vi "Calculate Feedforward.vi"() -> ()   [LabVIEW 2015]
uses:
  <vilib>/Rock Robotics/WPI/CAN/TalonSRX/WPI_CANTalonSRX_APIControlMode.ctl
  <vilib>/Rock Robotics/WPI/MotorControl/WPI_MotorControlOpenCANTalonSRX.vi
panel:
  in  "Counts per rev":i32
  in  "Device Number":i32
  in  "stop":bool
  in  "Start":bool
  in  "size of averaging array":i32
  in  "Deadzone":dbl format="%#_13g"
  out "Feedforward":dbl
  out "Applied Throttle":dbl
  out "Sensor Velocity":dbl
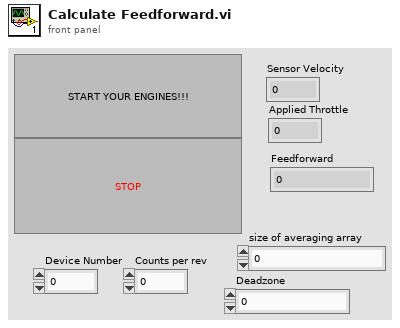
[diagram p1: front panel]
types:
  T1 = typedef "WPI_CANTalonSRX_APIControlMode.ctl" = enum8{"Percent VBus", "Speed", "Position", "Slave", "Unchanged / Invalid", "Voltage Compensation", "Current", "Motion Profile"}
  T2 = typedef "WPI_MotorControlDeviceRef.ctl" = cluster{"DeviceStatus":errorcluster, "Type":T3, "PWM":cluster{"PWM Channel":T4, "DeadBand":T5}, "CAN":cluster{"Device Number":u8, "Control Mode":T6, "Semaphore":T7, "Max Vout":dbl, "TalonSRX Control Mode":T1}, "Invert":bool}
  T3 = typedef "WPI_MotorControlType.ctl" = enum16{"PWM", "CAN", "CANTalonSRX"}
  T4 = typedef "FPGA_DIOPWMChannel.ctl" = enum8{"PWM 0", "PWM 1", "PWM 2", "PWM 3", "PWM 4", "PWM 5", "PWM 6", "PWM 7", "PWM 8", "PWM 9", "PWM MXP 0", "PWM MXP 1", "PWM MXP 2", "PWM MXP 3", "PWM MXP 4", "PWM MXP 5", "PWM MXP 6", "PWM MXP 7", "PWM MXP 8", "PWM MXP 9", "Invalid"}
  T5 = typedef "WPI_PWMDeadband.ctl" = cluster{"Name":string, "maxPositivePwm":i32, "minPositivePwm":i32, "centerPwm":i32, "maxNegativePwm":i32, "minNegativePwm":i32, "angularRange":u16}
  T6 = typedef "WPI_CANJaguar_ControlMode.ctl" = enum8{"Percent VBus", "Current", "Speed", "Position", "Voltage"}
  T7 = typedef "Semaphore RefNum" = refnum<k1>
  T8 = typedef "WPI_CANTalonSRX_GlobalStatus.ctl" = cluster{"Applied Throttle":dbl, "Module Enabled":bool, "CAN Error":errorcluster, "Closed Loop Error":dbl, "Forward Limit Switch Closed":bool, "Reverse Limit Switch Closed":bool, "Sensor Position":dbl, "Sensor Velocity":dbl, "Current":dbl, "Sticky Fault - Over Temp":bool, "Sticky Fault - Under Voltage":bool, "Sticky Fault - Forward Limit":bool, "Sticky Fault - Reverse Limit":bool, "Sticky Fault - Forward Soft Limit":bool, "Sticky Fault - Reverse Soft Limit":bool, "Brake is Enabled":bool, "Encoder Position":dbl, "Encoder Velocity":dbl, "Encoder Index Count":dbl, "Encoder A Pin State":bool, "Encoder B Pin State":bool, "Encoder Index Pin State":bool, "Analog In":dbl, "Analog In Velocity":dbl, "Temperature (C)":dbl, "Battery Voltage":dbl, "Control 5 Is Supported":bool, "Current Profile Slot Select":dbl, "Pos Div 8":bool, "Vel Div 4":bool, "Pulse Width Position":i32, "Pulse Width Velocity":i32, "Pulse Width Rise To Rise (us)":i32, "Pulse Width Rise To Fall (us)":i32, "Mot Prof Active Is Under Run":bool, "Mot Prof Active Has Under Run":bool, "Mot Prof Active Is Last":bool, "Mot Prof Active Velocity Only":bool, "Mot Prof Active Is Valid":bool, "Mot Prof Buffer Is Full":bool, "Mot Prof Active Profile Slot Select":i32, "Mot Prof NextID":i32, "Mot Prof Count":i32, "Mot Prof Active Velocity":dbl, "Mot Prof Active Position":dbl, "Mot Prof Output Enable":i32}
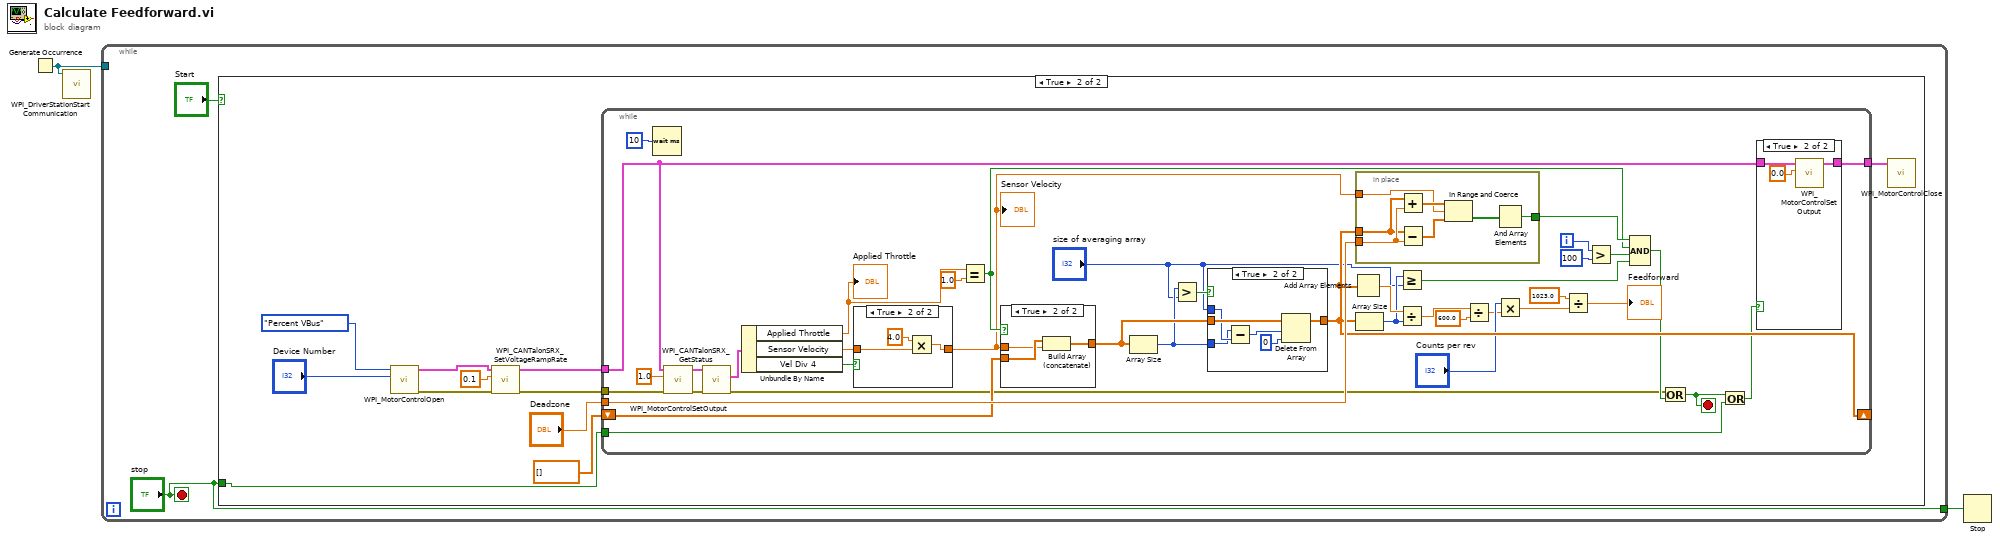
[diagram p0: block diagram]
diagram:
  n1 = Generate Occurrence() -> (w2:refnum<k4>)
  n2 = call <vilib>:"WPI_DriverStationStart Communication.vi"("occurrence"=w2) -> ()  [unwired: 1 in, 10 out]
  n3 = while {
    tunnel: w2 -> [_]
    tunnel: ["stop"] -> w1
    stop <- "stop" stop-if-true
    n4 = case shown="True" "Start" {
      tunnel: "stop" -> [_ w6]
      frame False {
      }
      frame True {
        n5 = call-poly <vilib>:"WPI_MotorControlOpen.vi"("Device Number"="Device Number", "Control Mode"=WPI_CANTalonSRX_APIControlMode."Percent VBus") -> ("error out"=w8:errorcluster, "MotorControlDeviceRef"=w11:T2)  [unwired: 8 in]
        n6 = call <vilib>:"WPI_CANTalonSRX_SetVoltageRampRate.vi"("error in (no error)"=w8, "Throttle Ramp Rate (percent/s)"=0.1, "CAN Talon SRX Ref"=w11) -> ("error out"=w7:errorcluster, "CAN Talon SRX Ref"=w10:T2)  [unwired: 7 in]
        n7 = while {
          tunnel: w10 -> [w45]
          tunnel: "Deadzone" -> [w53]
          shift-right: [w48] -> _
          shift-left: dbl[] [] -> [w52]
          tunnel: [w43] -> w9
          tunnel: w7 -> [w35]
          tunnel: w6 -> [w22]
          i -> [w42]
          stop <- w23 stop-if-true
          n8 = Wait (ms)(milliseconds to wait=u32 10) -> ()  [unwired: 1 out]
          n9 = call <vilib>:"WPI_MotorControlSetOutput.vi"("error in (no error)"=w35, "Output"=1.0, "MotorControlDevRef"=w45) -> ("error out"=w34:errorcluster, "MotorControlDevRef"=w44:T2)  [unwired: 6 in, 1 out]
          n10 = call <vilib>:"WPI_CANTalonSRX_GetStatus.vi"("error in (no error)"=w34, "CAN Talon SRX Ref"=w44) -> ("error out"=w33:errorcluster, "Talon SRX Status"=w54:T8)  [unwired: 7 in, 1 out]
          n11 = Unbundle By Name(w54) -> ("Applied Throttle"=w40:dbl, "Sensor Velocity"=w24:dbl, "Vel Div 4"=w26:bool)
          "Applied Throttle" <- w40
          n12 = case shown="True" w26 {
            tunnel: [w56 w57] -> w25
            tunnel: w24 -> [w56 w58]
            frame False {
            }
            frame True {
              n13 = Multiply(x=4.0, y=w58) -> (x*y=w57:dbl)
            }
          }
          "Sensor Velocity" <- w25
          n14 = Equal?(x=w40, y=1.0) -> (x = y?=w32:bool)
          n15 = case shown="True" w32 {
            tunnel: w52 -> [w67 w70]
            tunnel: [w67 w69] -> w50
            tunnel: w25 -> [_ w68]
            frame False {
            }
            frame True {
              n16 = Build Array (concatenate)(w70, w68) -> (w69:dbl[])
            }
          }
          n17 = Array Size(array=w50) -> (size(s)=w49:i32)
          n18 = Greater?(x=w49, y="size of averaging array") -> (0:w51:bool)
          n19 = case shown="True" w51 {
            tunnel: w50 -> [w75 w81]
            tunnel: "size of averaging array" -> [_ w80]
            tunnel: w49 -> [_ w79]
            tunnel: [w75 w76] -> w48
            frame False {
            }
            frame True {
              n20 = Subtract(x=w79, y=w80) -> (x-y=w78:i32)
              n21 = Delete From Array(array=w81, length=w78, index=0) -> (array with subset deleted=w76:dbl[])  [unwired: 1 out]
            }
          }
          n22 = Add Array Elements(numeric array=w48) -> (sum=w47:dbl)
          n23 = in-place {
            in-place-border: w53 -> [w64]
            in-place-border: w48 -> [w63]
            in-place-border: w25 -> [w62]
            in-place-border: [w60] -> w38
            n24 = Add(x=w63, y=w64) -> (x+y=w65:dbl[])
            n25 = Subtract(x=w63, y=w64) -> (x-y=w66:dbl[])
            n26 = In Range and Coerce(upper limit=w65, x=w62, lower limit=w66) -> (In Range?=w61:bool[])  [unwired: 1 out]
            n27 = And Array Elements(Boolean array=w61) -> (logical AND=w60:bool)
          }
          n28 = Array Size(array=w48) -> (size(s)=w29:i32)
          n29 = Greater Or Equal?(x=w29, y="size of averaging array") -> (x >= y?=w27:bool)
          n30 = Divide(x=w47, y=w29) -> (x/y=w20:dbl)
          n31 = Divide(x=w20, y=600.0) -> (x/y=w17:dbl)
          n32 = Multiply(x="Counts per rev", y=w17) -> (x*y=w16:dbl)
          n33 = Divide(x=1023.0, y=w16) -> (x/y=→"Feedforward":dbl)
          n34 = Greater?(x=w42, y=100) -> (0:w37:bool)
          n35 = Compound Arithmetic op=AND(w38, w32, w37, w27) -> (w36:bool)
          n36 = Or(x=w33, y=w36) -> (x .or. y?=w23:bool)
          n37 = Or(x=w23, y=w22) -> (x .or. y?=w21:bool)
          n38 = case shown="True" w21 {
            tunnel: w45 -> [w71 w73]
            tunnel: [w71 w72] -> w43
            frame False {
            }
            frame True {
              n39 = call <vilib>:"WPI_MotorControlSetOutput.vi"("Output"=0.0, "MotorControlDevRef"=w73) -> ("MotorControlDevRef"=w72:T2)  [unwired: 7 in, 2 out]
            }
          }
        }
        n40 = call <vilib>:"WPI_MotorControlClose.vi"("MotorControlDevRef"=w9) -> ()  [unwired: 10 in, 1 out]
      }
    }
  }
  n41 = Stop(stop? (T)=w1) -> ()
